vi "DBM Unit Set.vi"(7 "분류코드":string, 8 "에러 입력(에러 없음)":errorcluster, 9 "교정기능 문자열[]":string[](array[string]), 11 "참조":T1) -> (0 "에러 출력":errorcluster, 3 "SQL query 컬럼명":string, 4 "Condition2 캡션":string)   [LabVIEW 2020]
uses:
  Variables/Global_Constant.vi
  Public/Polymorph/Rmv Empt Arr_1D Str.vi
  Public/Polymorph/Cell Space_Table.vi
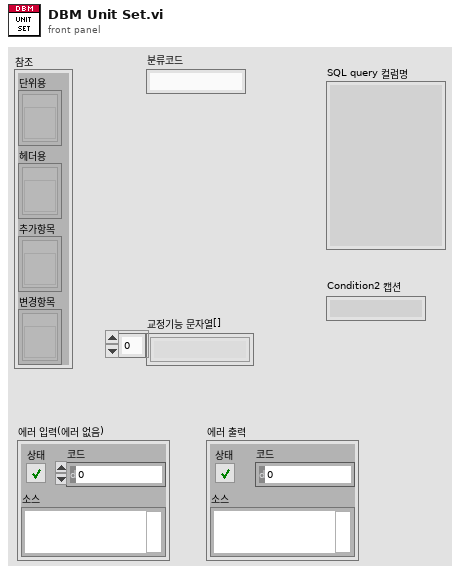
[diagram p1: front panel]
types:
  T1 = cluster{"단위용":refnum<vi>[], "헤더용":refnum<vi>[], "추가항목":refnum<vi>[], "변경항목":refnum<vi>[]}
  T2 = cluster{"구분 1 캡션":string, "구분 1 리스트":string[], "구분 2 캡션":string, "구분 2 리스트":string[]}
  T3 = cluster{"Display sys":string[], "변경항목비활성":i32[], "추가항목비활성":i32[]}
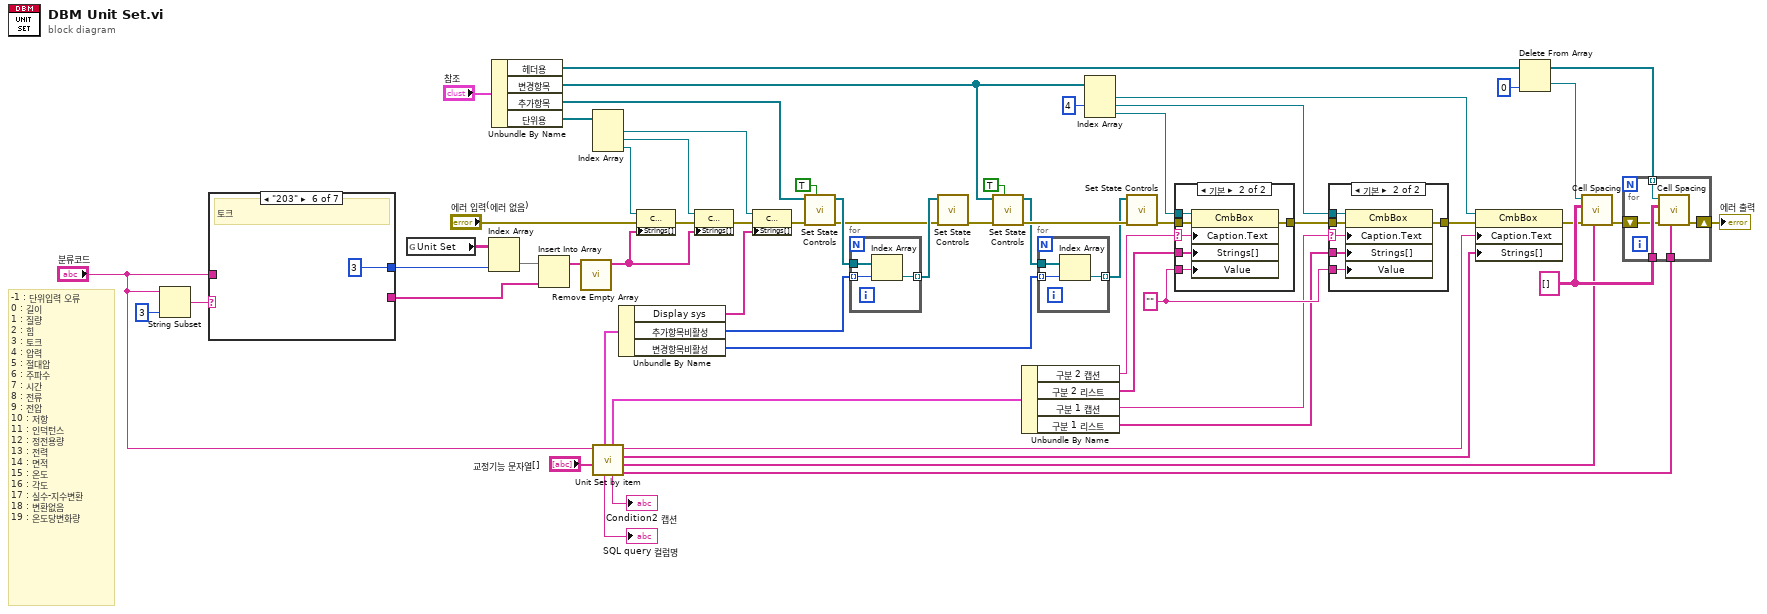
[diagram p0: block diagram]
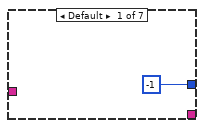
[diagram p4: hidden frame]
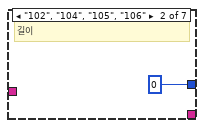
[diagram p5: hidden frame]
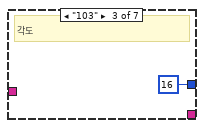
[diagram p6: hidden frame]
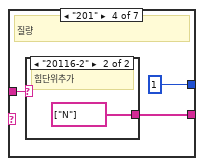
[diagram p7: hidden frame]
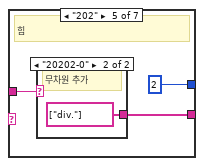
[diagram p9: hidden frame]
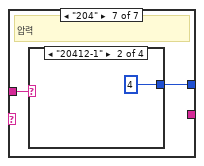
[diagram p11: hidden frame]
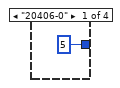
[diagram p12: hidden frame]
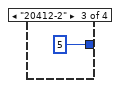
[diagram p13: hidden frame]
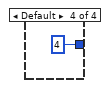
[diagram p14: hidden frame]
diagram:
  w38 = "" ("값")
  w56 = string[][] [] ("Data in")
  # "-1 : 단위입력 오류\n0 : 길이\n1 : 질량\n2 : 힘\n3 : 토크\n4 : 압력\n5 : 절대압\n6 : 주파수\n7 : 시간\n8 : 전류\n9 : 전압\n10 : 저항\n11 : 인덕턴스\n12 : 정전용량 \n13 : 전력\n14 : 면적\n15 : 온도\n16 : 각도\n17 : 실수-지수변환\n18 : 변환없음\n19 : 온도당변화량"
  n1 = String Subset(string="분류코드", length (rest)=3 ("길이(나머지)")) -> (substring=w59:string)  [unwired: 1 in]
  n2 = case shown="\"203\"" w59 {
    tunnel: [-1 ("비활성화된 인덱스 (열)") 0 ("비활성화된 인덱스 (열)") 16 ("비활성화된 인덱스 (열)") 1 ("비활성화된 인덱스 (열)") 2 ("비활성화된 인덱스 (열)") 3 ("비활성화된 인덱스 (열)") w75] -> w61
    tunnel: "분류코드" -> [_ _ _ w66 w69 _ w74]
    tunnel: [_ _ _ w65 w70 _ _] -> w45
    frame Default {
    }
    frame "102", "104", "105", "106" {
      # "길이"
    }
    frame "103" {
      # "각도"
    }
    frame "201" {
      # "질량"
      n3 = case shown="\"20116-2\"" w66 {
        tunnel: [_ string[] ["N"]] -> w65
        frame Default {
        }
        frame "20116-2" {
          # "힘단위추가"
        }
      }
    }
    frame "202" {
      # "힘"
      n4 = case shown="\"20202-0\"" w69 {
        tunnel: [_ string[] ["div."] ("Unit Set")] -> w70
        frame Default {
        }
        frame "20202-0" {
          # "무차원 추가"
        }
      }
    }
    frame "203" {
      # "토크"
    }
    frame "204" {
      # "압력"
      n5 = case shown="\"20412-1\"" w74 {
        tunnel: [5 ("비활성화된 인덱스 (열)") 4 ("비활성화된 인덱스 (열)") 5 ("비활성화된 인덱스 (열)") 4 ("비활성화된 인덱스 (열)")] -> w75
        frame "20406-0" {
        }
        frame "20412-1" {
        }
        frame "20412-2" {
        }
        frame Default {
        }
      }
    }
  }
  n6 = global read "Global_Constant.vi" "Unit Set"() -> (w55:string[][])
  n7 = Index Array(array=w55, index (col)=w61) -> (element=w46:string[])  [unwired: 1 in]
  n8 = Unbundle By Name("참조") -> ("헤더용"=w23:refnum<vi>[], "변경항목"=w22:refnum<vi>[], "추가항목"=w15:refnum<vi>[], "단위용"=w24:refnum<vi>[])
  n9 = Insert Into Array(array=w46, new element=w45) -> (w44:string[])  [unwired: 1 in]
  n10 = call-poly "Remove Empty Array.vi"("Data in"=w44) -> ("Data out"=w47:string[])  [unwired: 9 in, 1 out]
  n11 = Index Array(array=w24) -> (element #1=w58:refnum<vi>, element #2=w48:refnum<vi>, element #3=w49:refnum<vi>)  [unwired: 3 in]
  n12 = call "Unit Set by item.vi"("교정기능 2 리스트"="교정기능 문자열[]", "분류코드"="분류코드") -> ("컬럼 헤더+CMC"=w12:string[], "컬럼 헤더"=w11:string[], "교정기능 2 리스트 2"=w5:string[], "교정기능 2 캡션"=w4:string, "Condition2 캡션"=→"Condition2 캡션":string, "콤보박스"=w3:T2, "SQL query"=→"SQL query 컬럼명":string, "클러스터"=w30:T3)  [unwired: 2 in]
  n13 = Unbundle By Name(w30) -> ("Display sys"=w34:string[], "추가항목비활성"=w14:i32[], "변경항목비활성"=w29:i32[])
  n14 = property on="프로퍼티 노드" class="CmbBox"(reference=w49, error in="에러 입력(에러 없음)", "Strings[]"=w47) -> (error out=w51:errorcluster)  [unwired: 1 out]
  n15 = property on="프로퍼티 노드" class="CmbBox"(reference=w48, error in=w51, "Strings[]"=w47) -> (error out=w50:errorcluster)  [unwired: 1 out]
  n16 = property on="프로퍼티 노드" class="CmbBox"(reference=w58, error in=w50, "Strings[]"=w34) -> (error out=w16:errorcluster)  [unwired: 1 out]
  n17 = call "Set State Controls.vi"("활성화 (F)"=TRUE, "error in (no error)"=w16, "컨트롤 참조 배열 in"=w15) -> ("error out"=w40:errorcluster, "컨트롤 참조 배열 out"=w41:refnum<vi>[])  [unwired: 7 in]
  n18 = for {
    tunnel: w14 -> [w81] mode=indexing
    tunnel: w41 -> [w82]
    tunnel: [w80] -> w42 mode=indexing
    n19 = Index Array(array=w82, index=w81) -> (element=w80:refnum<vi>)
  }
  n20 = call "Set State Controls.vi"("error in (no error)"=w40, "컨트롤 참조 배열 in"=w42) -> ("error out"=w13:errorcluster)  [unwired: 8 in, 1 out]
  n21 = call "Set State Controls.vi"("활성화 (F)"=TRUE, "error in (no error)"=w13, "컨트롤 참조 배열 in"=w22) -> ("error out"=w54:errorcluster, "컨트롤 참조 배열 out"=w53:refnum<vi>[])  [unwired: 7 in]
  n22 = Unbundle By Name(w3) -> ("구분 2 캡션"=w9:string, "구분 2 리스트"=w8:string[], "구분 1 캡션"=w33:string, "구분 1 리스트"=w32:string[])
  n23 = for {
    tunnel: w29 -> [w84] mode=indexing
    tunnel: w53 -> [w85]
    tunnel: [w83] -> w52 mode=indexing
    n24 = Index Array(array=w85, index=w84) -> (element=w83:refnum<vi>)
  }
  n25 = Index Array(array=w22, index #2=4 ("인덱스")) -> (element #1=w26:refnum<vi>, element #2=w18:refnum<vi>, element #3=w17:refnum<vi>)  [unwired: 2 in]
  n26 = call "Set State Controls.vi"("error in (no error)"=w54, "컨트롤 참조 배열 in"=w52) -> ("error out"=w10:errorcluster)  [unwired: 8 in, 1 out]
  n27 = case shown="기본" w9 {
    selector: w9 -> [_ w91]
    tunnel: w17 -> [_ w92]
    tunnel: w8 -> [_ w90]
    tunnel: w38 -> [_ w89]
    tunnel: w10 -> [w86 w88]
    tunnel: [w86 w87] -> w7
    frame "" {
    }
    frame Default {
      n28 = property on="프로퍼티 노드" class="CmbBox"(reference=w92, error in=w88, "Caption.Text"=w91, "Strings[]"=w90, "Value"=w89) -> (error out=w87:errorcluster)  [unwired: 1 out]
    }
  }
  n29 = case shown="기본" w33 {
    selector: w33 -> [_ w98]
    tunnel: w18 -> [_ w99]
    tunnel: w32 -> [_ w97]
    tunnel: w38 -> [_ w96]
    tunnel: w7 -> [w93 w95]
    tunnel: [w93 w94] -> w6
    frame "" {
    }
    frame Default {
      n30 = property on="프로퍼티 노드" class="CmbBox"(reference=w99, error in=w95, "Caption.Text"=w98, "Strings[]"=w97, "Value"=w96) -> (error out=w94:errorcluster)  [unwired: 1 out]
    }
  }
  n31 = property on="프로퍼티 노드" class="CmbBox"(reference=w26, error in=w6, "Caption.Text"=w4, "Strings[]"=w5) -> (error out=w2:errorcluster)  [unwired: 1 out]
  n32 = Delete From Array(array=w23, index=0 ("인덱스")) -> (deleted portion=w36:refnum<vi>, array with subset deleted=w35:refnum<vi>[])  [unwired: 1 in]
  n33 = call-poly "Cell Spacing.vi"("Col Header in"=w11, "error in"=w2, "Data in"=w56, "테이블 참조 in"=w36) -> ("error out"=w21:errorcluster)  [unwired: 5 in, 2 out]
  n34 = for {
    tunnel: w56 -> [w103]
    tunnel: w12 -> [w102]
    shift-right: [w104] -> w20
    shift-left: w21 -> [w101]
    tunnel: w35 -> [w100] mode=indexing
    n35 = call-poly "Cell Spacing.vi"("Col Header in"=w102, "error in"=w101, "Data in"=w103, "테이블 참조 in"=w100) -> ("error out"=w104:errorcluster)  [unwired: 5 in, 2 out]
  }
  "에러 출력" <- w20
